vi "validate_ManipJump_v0.01.vi"(0 "Start Position":T3(ring), 1 "which manipulator":T5(ring), 2 "valve Time Cluster":T2, 3 "data in":T4={"daq_ao 1"="Dev1/ao0", "daq_ai 1"="Dev1/ai0", "experiment day folder"=path "D:/DATA/8-27-15 save func testing/test.lvm", "Multiclamp init error"=0, "Multiclamp Handle Out"=0, "sampling rate (Hz)"=10000, "trial name"=""}, 5 "Jump Position":T3(ring), 7 "controls array in":refnum<vi>[](array[refnum]), 9 "time to wait for solution change (min)":dbl=2.5 min=0.0 step=0.01, 11 "error in":errorcluster, 12 "common cluster":T7, 13 "individual controls in":T6) -> (4 "output cluster":T1={"daq_ao 2"="", "Duration (s)"=0.0, "Sample Freq (Hz)"=0.0, "Phase"=0.0, "Duty Cycle"=0.0, "Jump Filter Freq (Hz)"=0.0, "Number of Replicates"=1} {"Number of Replicates" min=1 max=10}, 6 "protocol waveform":waveform(dbl)(graph), 8 "protocol response":waveform(dbl)[](graph) caption="protcol response", 10 "control array out":refnum<vi>[](array[refnum]), 15 "error out":errorcluster)   [LabVIEW 2019]
uses:
  controls/scope_motion.ctl
  pipette cleaning/pressure box/cleaning_soft/controls/actuator_type.ctl
  pipette cleaning/pressure box/cleaning_soft/controls/actuator_cluster.ctl
  machine_vision/coordinate model vis/transform_properties_actuators.ctl
  machine_vision/controls/transform_cluster_actuator.ctl
  controls/NH_method.ctl
  pipette cleaning/pressure box/cleaning_soft/controls/pressure_box_type.ctl
  pipette cleaning/pressure box/cleaning_soft/controls/pressure_box_control.ctl
  multipatch/controls/multipatch_common_controls_v4.ctl
  controls/memtest_def.ctl
  multipatch/controls/multipatch_individual_controls_v5.ctl
  Controls/Data.ctl
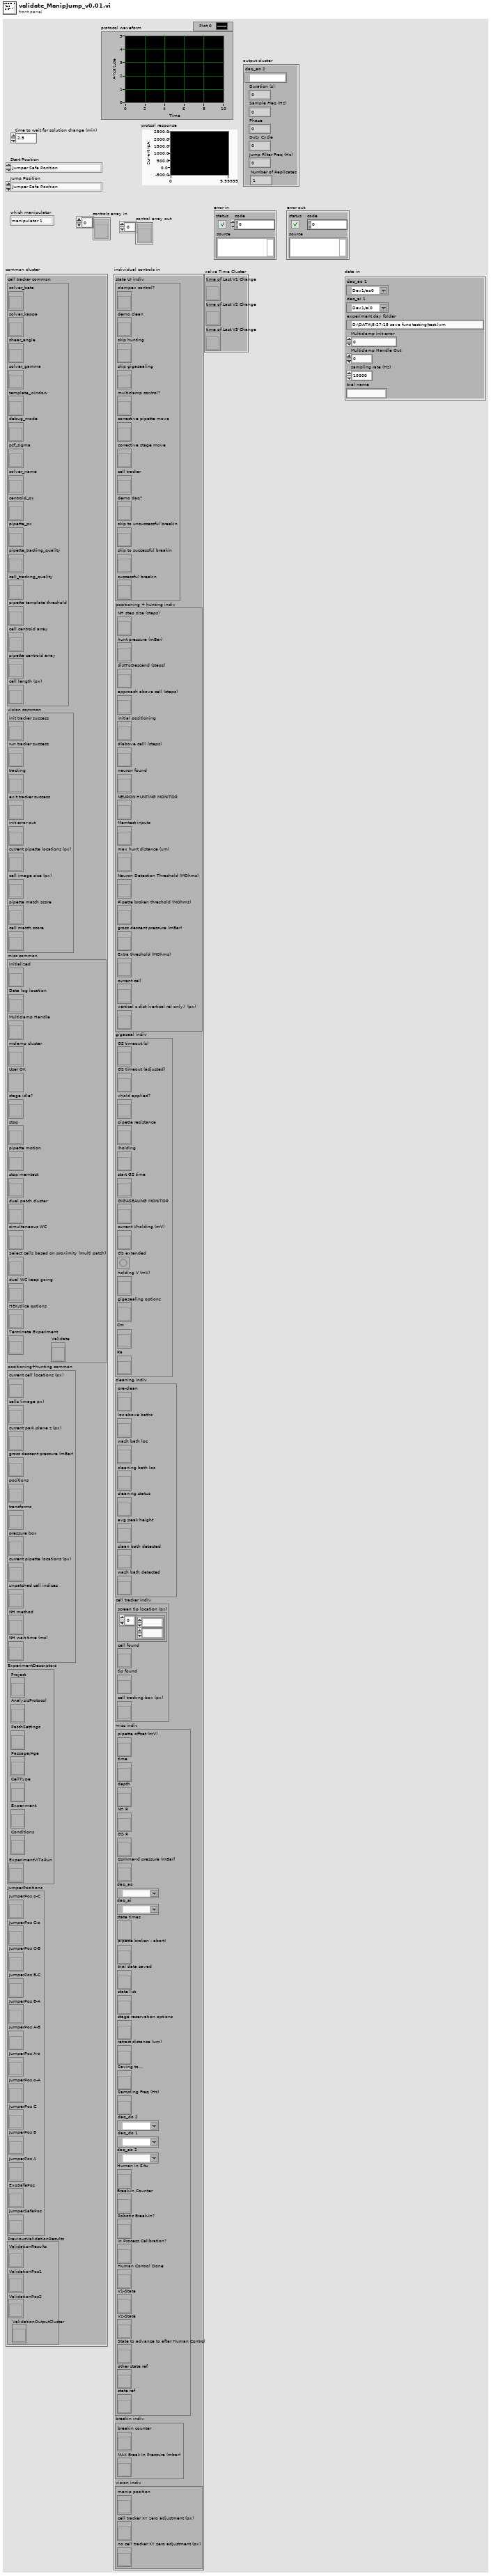
[diagram p1: front panel]
types:
  T1 = cluster{"daq_ao 2":tag, "Duration (s)":dbl, "Sample Freq (Hz)":dbl, "Phase":dbl, "Duty Cycle":dbl, "Jump Filter Freq (Hz)":dbl, "Number of Replicates":i16}
  T2 = cluster{"time of Last V1 Change":refnum<vi>, "time of Last V2 Change":refnum<vi>, "time of Last V3 Change":refnum<vi>}
  T3 = enum16{"Jumper Safe Position", "Experiment Safe Position", "Jumper Position A", "Jumper Position B", "Jumper Position C", "Jumper Position o-A", "Jumper Position A-o", "Jumper Position A-B", "Jumper Position B-A", "Jumper Position B-C", "Jumper Position C-B", "Jumper Position C-o", "Jumper Position o-C"}
  T4 = typedef "Data.ctl" = cluster{"daq_ao 1":tag, "daq_ai 1":tag, "experiment day folder":path, "Multiclamp init error":i32, "Multiclamp Handle Out":u32, "sampling rate (Hz)":i32, "trial name":string}
  T5 = enum16{"manipulator 1", "manipulator 2", "manipulator 3", "manipulator 4"}
  T6 = typedef "multipatch_individual_controls_v5.ctl" = cluster{"state UI indiv":cluster{"clampex control?":refnum<vi>, "demo clean":refnum<vi>, "skip hunting":refnum<vi>, "skip gigasealing":refnum<vi>, "multiclamp control?":refnum<vi>, "corrective pipette move":refnum<vi>, "corrective stage move":refnum<vi>, "cell tracker":refnum<vi>, "demo daq?":refnum<vi>, "skip to unsuccessful breakin":refnum<vi>, "skip to successful breakin":refnum<vi>, "successful breakin":refnum<vi>}, "positioning + hunting indiv":cluster{"NH step size (steps)":refnum<vi>, "hunt pressure (mBar)":refnum<vi>, "distToDescend (steps)":refnum<vi>, "approach above cell (steps)":refnum<vi>, "initial positioning":refnum<vi>, "d(above cell) (steps)":refnum<vi>, "neuron found":refnum<vi>, "NEURON HUNTING MONITOR":refnum<vi>, "Memtest inputs":refnum<vi>, "max hunt distance (um)":refnum<vi>, "Neuron Detection Threshold (MOhms)":refnum<vi>, "Pipette broken threshold (MOhms)":refnum<vi>, "gross descent pressure (mBar)":refnum<vi>, "Extra threshold (MOhms)":refnum<vi>, "current cell":refnum<vi>, "vertical z dist (vertical rel only)  (px)":refnum<vi>}, "gigaseal indiv":cluster{"GS timeout (s)":refnum<vi>, "GS timeout (adjusted)":refnum<vi>, "vhold applied?":refnum<vi>, "pipette resistance":refnum<vi>, "Iholding":refnum<vi>, "start GS time":refnum<vi>, "GIGASEALING MONITOR":refnum<vi>, "current Vholding (mV)":refnum<vi>, "GS extended":refnum<vi>, "holding V (mV)":refnum<vi>, "gigasealing options":refnum<vi>, "Cm":refnum<vi>, "Ra ":refnum<vi>}, "cleaning indiv":cluster{"pre-clean":refnum<vi>, "loc above baths":refnum<vi>, "wash bath loc":refnum<vi>, "cleaning bath loc":refnum<vi>, "cleaning status":refnum<vi>, "avg peak height":refnum<vi>, "clean bath detected":refnum<vi>, "wash bath detected":refnum<vi>}, "cell tracker indiv":cluster{"screen tip location (px)":refnum<vi>, "cell found":refnum<vi>, "tip found":refnum<vi>, "cell tracking box (px)":refnum<vi>}, "misc indiv":cluster{"pipette offset (mV)":refnum<vi>, "time":refnum<vi>, "depth":refnum<vi>, "NH R":refnum<vi>, "GS R":refnum<vi>, "Command pressure (mBar)":refnum<vi>, "daq_ao":tag, "daq_ai":tag, "state times":refnum<vi>, "pipette broken - abort!":refnum<vi>, "trial data saved":refnum<vi>, "state list":refnum<vi>, "stage reservation options":refnum<vi>, "retract distance (um)":refnum<vi>, "Saving to...":refnum<vi>, "Sampling Freq (Hz)":refnum<vi>, "daq_do 2":tag, "daq_do 1":tag, "daq_ao 2":tag, "Human in Situ":refnum<vi>, "Break-In Counter":refnum<vi>, "Robotic Break-In?":refnum<vi>, "In Process Calibration?":refnum<vi>, "Human Control Done":refnum<vi>, "V1-State":refnum<vi>, "V2-State":refnum<vi>, "State to advance to after Human Control":refnum<vi>, "other state ref":refnum<vi>, "state ref":refnum<vi>}, "breakin indiv":cluster{"breakin counter":refnum<vi>, "MAX Break In Pressure (mbar)":refnum<vi>}, "vision indiv":cluster{"manip position":refnum<vi>, "cell tracker XY zero adjustment (px)":refnum<vi>, "no cell tracker XY zero adjustment (px)":refnum<vi>}}
  T7 = typedef "multipatch_common_controls_v4.ctl" = cluster{"cell tracker common":cluster{"solver_beta":refnum<vi>, "solver_kappa":refnum<vi>, "shear_angle":refnum<vi>, "solver_gamma":refnum<vi>, "template_window":refnum<vi>, "debug_mode":refnum<vi>, "psf_sigma":refnum<vi>, "solver_name":refnum<vi>, "centroid_px":refnum<vi>, "pipette_px":refnum<vi>, "pipette_tracking_quality":refnum<vi>, "cell_tracking_quality":refnum<vi>, "pipette template threshold":refnum<vi>, "cell centroid array":refnum<vi>, "pipette centroid array":refnum<vi>, "cell length (px)":refnum<vi>}, "vision common":cluster{"init tracker success":refnum<vi>, "run tracker success":refnum<vi>, "tracking":refnum<vi>, "exit tracker success":refnum<vi>, "init error out":refnum<vi>, "current pipette locations (px)":refnum<vi>, "cell image size (px)":refnum<vi>, "pipette match score":refnum<vi>, "cell match score":refnum<vi>}, "misc common":cluster{"initialized":refnum<vi>, "Data log location":refnum<vi>, "Multiclamp Handle":refnum<vi>, "mclamp cluster":refnum<vi>, "User OK":refnum<vi>, "stage idle?":refnum<vi>, "stop":refnum<vi>, "pipette motion":refnum<vi>, "stop memtest":refnum<vi>, "dual patch cluster":refnum<vi>, "simultaneous WC":refnum<vi>, "Select cells based on proximity (multi patch)":refnum<vi>, "dual WC keep going":refnum<vi>, "HEK/slice options":refnum<vi>, "Terminate Experiment":refnum<vi>, "Validate":refnum<vi>}, "positioning+hunting common":cluster{"current cell locations (px)":refnum<vi>, "cells (image px)":refnum<vi>, "current park plane z (px)":refnum<vi>, "gross descent pressure (mBar)":refnum<vi>, "positions":refnum<vi>, "transforms":refnum<vi>, "pressure box":refnum<vi>, "current pipette locations (px)":refnum<vi>, "unpatched cell indices":refnum<vi>, "NH method":refnum<vi>, "NH wait time (ms)":refnum<vi>}, "ExperimentDescriptors":cluster{"Project":refnum<vi>, "AnalysisProtocol":refnum<vi>, "PatchSettings":refnum<vi>, "Passage/Age":refnum<vi>, "CellType":refnum<vi>, "Experiment":refnum<vi>, "Conditions":refnum<vi>, "ExperimentVIToRun":refnum<vi>}, "JumperPositions":cluster{"JumperPos o-C":refnum<vi>, "JumperPos C-o":refnum<vi>, "JumperPos C-B":refnum<vi>, "JumperPos B-C":refnum<vi>, "JumperPos B-A":refnum<vi>, "JumperPos A-B":refnum<vi>, "JumperPos A-o":refnum<vi>, "JumperPos o-A":refnum<vi>, "JumperPos C":refnum<vi>, "JumperPos B":refnum<vi>, "JumperPos A":refnum<vi>, "ExpSafePos":refnum<vi>, "jumperSafePos":refnum<vi>}, "PreviousValidationResults":cluster{"ValidationResults":refnum<vi>, "ValidationPos1":refnum<vi>, "ValidationPos2":refnum<vi>, "ValidationOutputCluster":refnum<vi>}}
  T8 = typedef "transform_cluster_actuator.ctl" = cluster{"s":refnum<vi>, "manip 1":refnum<vi>, "manip 2":refnum<vi>, "manip 3":refnum<vi>, "manip 4":refnum<vi>}
  T9 = typedef "scope_motion.ctl" = enum16{"superSlow", "fast", "slow", "find slice speed", "slow_dualPatch"}
  T10 = typedef "transform_properties_actuators.ctl" = cluster{"theta (deg)":dbl, "X sc factor (px/step)":dbl, "Y sc factor (px/step)":dbl, "zero loc (x,y,z)":dbl[], "flip y?":bool, "flip x?":bool, "gamma (deg)":dbl, "flip z?":bool, "Z sc factor (px/step)":dbl, "actuator":T11, "safe space (steps)":i32[]}
  T11 = typedef "actuator_cluster.ctl" = cluster{"Actuator COM":refnum<visa-resource-name>, "Actuator type":T12}
  T12 = typedef "actuator_type.ctl" = enum16{"Scientifica", "Sutter", "Demo", "Off"}
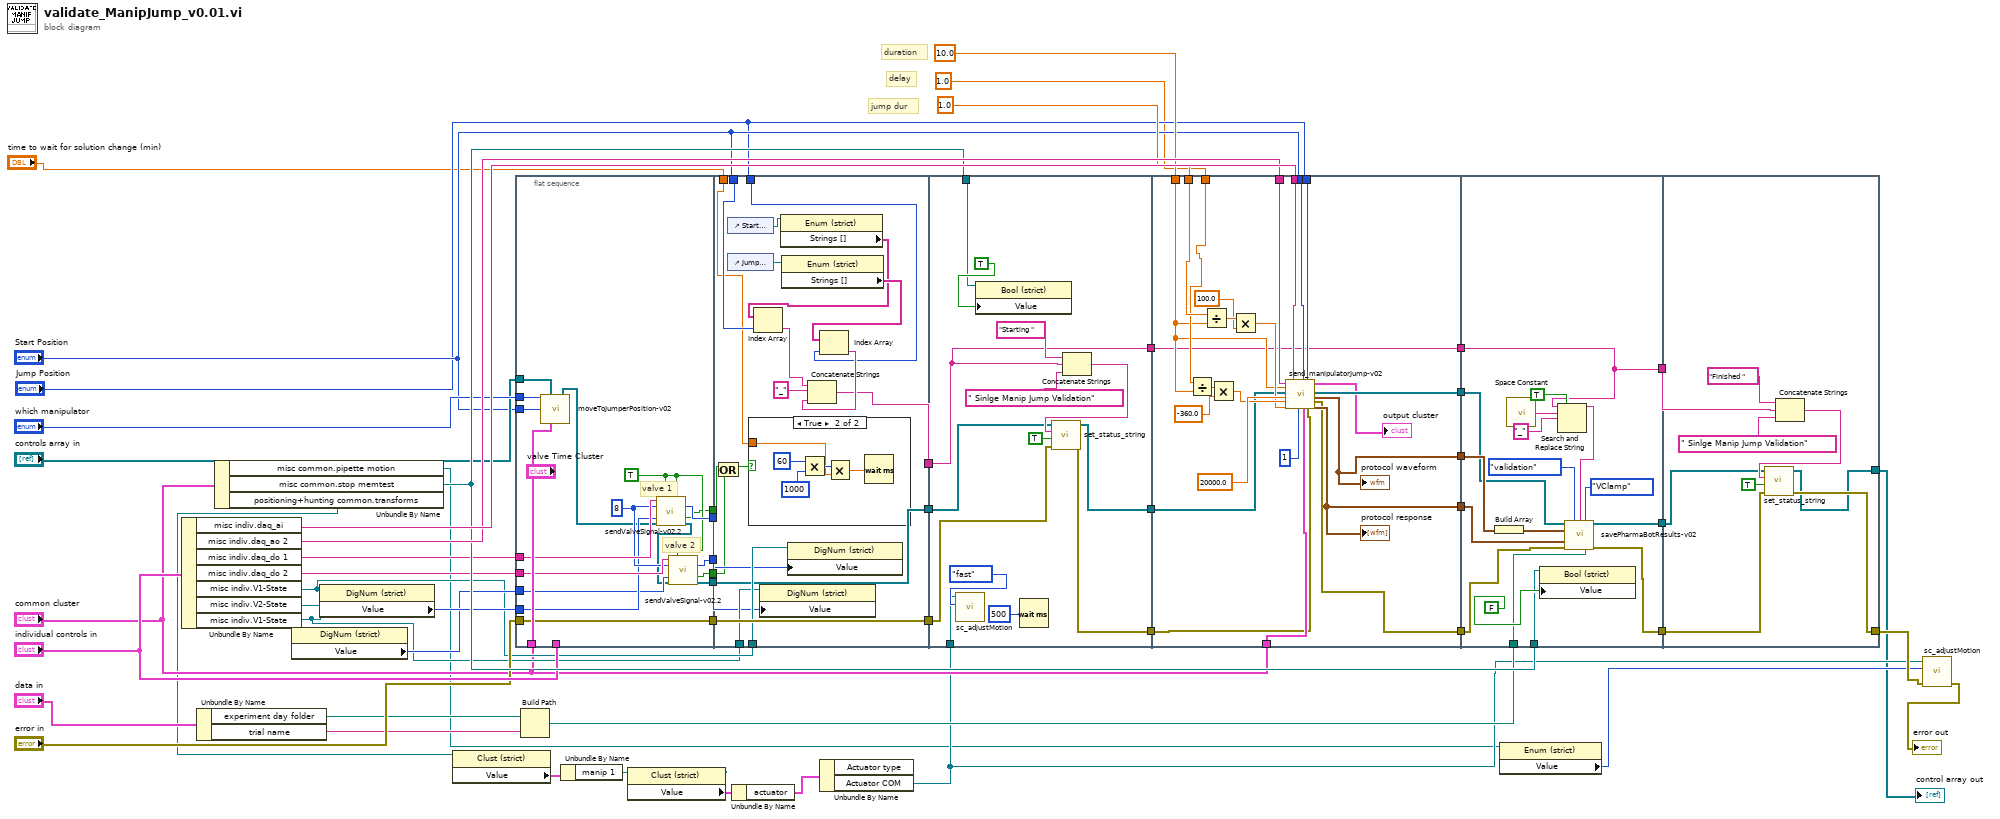
[diagram p0: block diagram]
diagram:
  # "jump dur"
  # "delay"
  # "duration"
  n1 = Unbundle By Name("individual controls in") -> ("misc indiv.daq_ai"=w55:tag, "misc indiv.daq_ao 2"=w54:tag, "misc indiv.daq_do 1"=w50:tag, "misc indiv.daq_do 2"=w49:tag, "misc indiv.V1-State"=w41:refnum<vi>, "misc indiv.V2-State"=w40:refnum<vi>)  [unwired: 1 out]
  n2 = Unbundle By Name("data in") -> ("experiment day folder"=w34:path, "trial name"=w33:string)
  n3 = Unbundle By Name("common cluster") -> ("misc common.pipette motion"=w21:refnum<vi>, "misc common.stop memtest"=w53:refnum<vi>, "positioning+hunting common.transforms"=w28:refnum<vi>)
  n4 = property class="DigNum (strict)"(reference=w40) -> ("Value"=w42:u16)  [unwired: 1 in, 2 out]
  n5 = property class="DigNum (strict)"(reference=w41) -> ("Value"=w43:u16)  [unwired: 1 in, 2 out]
  n6 = property class="Clust (strict)"(reference=w28) -> ("Value"=w29:T8)  [unwired: 1 in, 2 out]
  n7 = flat-sequence {
    tunnel: "which manipulator" -> [w73]
    tunnel: "Start Position" -> [w72]
    tunnel: "common cluster" -> [w71]
    tunnel: "individual controls in" -> [_]
    tunnel: w50 -> [w70]
    tunnel: w49 -> [w69]
    tunnel: "error in" -> [w67]
    tunnel: [w67] -> w44
    tunnel: w43 -> [w66]
    tunnel: w42 -> [w65]
    tunnel: [w64] -> w39
    tunnel: [w63] -> w38
    tunnel: "controls array in" -> [w62]
    tunnel: [w59] -> w15
    tunnel: [w57] -> w3
    tunnel: [w56] -> w2
    tunnel: [w93] -> w45
    tunnel: w44 -> [w93]
    tunnel: w41 -> [w92]
    tunnel: w40 -> [w91]
    tunnel: w39 -> [w90]
    tunnel: w38 -> [w89]
    tunnel: [w88] -> w16
    tunnel: w15 -> [w88]
    tunnel: "Start Position" -> [w80]
    tunnel: "Jump Position" -> [w79]
    tunnel: [w78] -> w7
    tunnel: w3 -> [w76]
    tunnel: w2 -> [w75]
    tunnel: "time to wait for solution change (min)" -> [w74]
    tunnel: w53 -> [w110]
    tunnel: [w99] -> w46
    tunnel: w45 -> [w100]
    tunnel: w23 -> [w108]
    tunnel: w16 -> [w102]
    tunnel: [w101] -> w14
    tunnel: w7 -> [w103]
    tunnel: [w103] -> w5
    tunnel: w55 -> [w135]
    tunnel: w54 -> [w134]
    tunnel: [w118] -> w47
    tunnel: w46 -> [w119]
    tunnel: [w114] -> w37
    tunnel: [w133] -> w36
    tunnel: "common cluster" -> [w120]
    tunnel: "Start Position" -> [w132]
    tunnel: "Jump Position" -> [w131]
    tunnel: 10.0 ("Duration (s)") -> [w121]
    tunnel: 1.0 ("Jump Duration (s)") -> [w126]
    tunnel: 1.0 ("Jump Delay (s)") -> [w125]
    tunnel: w14 -> [w117]
    tunnel: [w116] -> w13
    tunnel: [w115] -> w6
    tunnel: w5 -> [w115]
    tunnel: w53 -> [w152]
    tunnel: w47 -> [w141]
    tunnel: w37 -> [w151]
    tunnel: w36 -> [w149]
    tunnel: w32 -> [w146]
    tunnel: [w137] -> w18
    tunnel: w13 -> [w140]
    tunnel: [w139] -> w12
    tunnel: [w138] -> w10
    tunnel: w6 -> [w138]
    tunnel: [w157] -> w25
    tunnel: w18 -> [w158]
    tunnel: w12 -> [w159]
    tunnel: [w156] -> w11
    tunnel: w10 -> [w155]
    frame #0 {
      w58 = TRUE ("Set Status")
      w68 = u16 8 ("ChangeToValve")
      # "valve 2"
      # "valve 1"
      n8 = call "moveToJumperPosition-v02.vi"("which manipulator"=w73, "controls array in"=w62, "Which Jumper Position to move to?"=w72, "common cluster"=w71) -> ("control array out"=w61:refnum<vi>[])  [unwired: 10 in, 1 out]
      n9 = call "sendValveSignal-v02.2.vi"("daq_do"=w70, "Valve1?"=w58, "ChangeToValve"=w68, "CurrentValve"=w66, "controls array in"=w61, "Set Status"=w58) -> ("ValveSetTo"=w63:u16, "valve changed?"=w57:bool, "control array out"=w60:refnum<vi>[])  [unwired: 6 in, 1 out]
      n10 = call "sendValveSignal-v02.2.vi"("daq_do"=w69, "ChangeToValve"=w68, "CurrentValve"=w65, "controls array in"=w60, "Set Status"=w58) -> ("ValveSetTo"=w64:u16, "valve changed?"=w56:bool, "control array out"=w59:refnum<vi>[])  [unwired: 7 in, 1 out]
    }
    frame #1 {
      n11 = Or(x=w76, y=w75) -> (x .or. y?=w77:bool)
      n12 = control-ref of="Start Position"() -> (w82:refnum<vi>)
      n13 = control-ref of="Jump Position"() -> (w83:refnum<vi>)
      n14 = case shown="True" w77 {
        tunnel: w74 -> [_ w94]
        frame False {
        }
        frame True {
          n15 = Multiply(x=u32 60 ("milliseconds to wait"), y=u32 1000) -> (x*y=w96:u32)
          n16 = Multiply(x=w96, y=w94) -> (x*y=w95:dbl)
          n17 = Wait (ms)(milliseconds to wait=w95) -> ()  [unwired: 1 out]
        }
      }
      n18 = property class="DigNum (strict)"(reference=w91, "Value"=w90) -> ()  [unwired: 1 in, 2 out]
      n19 = property class="Enum (strict)"(reference=w82) -> ("Strings []"=w86:string[])  [unwired: 1 in, 2 out]
      n20 = Index Array(array=w86, index=w80) -> (element=w85:string)
      n21 = property class="Enum (strict)"(reference=w83) -> ("Strings []"=w87:string[])  [unwired: 1 in, 2 out]
      n22 = property class="DigNum (strict)"(reference=w92, "Value"=w89) -> ()  [unwired: 1 in, 2 out]
      n23 = Index Array(array=w87, index=w79) -> (element=w81:string)
      n24 = Concatenate Strings(w85, "_", w81) -> (w78:string)
    }
    frame #2 {
      n25 = call "sc_adjustMotion.vi"("motion"=scope_motion."fast", "VISA handle"=w108) -> ()  [unwired: 8 in, 2 out]
      n26 = property class="Bool (strict)"(reference=w110, "Value"=TRUE ("stop memtest")) -> ()  [unwired: 1 in, 2 out]
      n27 = Wait (ms)(milliseconds to wait=u32 500) -> ()  [unwired: 1 out]
      n28 = Concatenate Strings("Starting " ("string"), w103, " Sinlge Manip Jump Validation" ("string")) -> (w106:string)
      n29 = call "set_status_string.vi"("error in"=w100, "new line?"=TRUE, "status string in"=w106, "controls array"=w102) -> ("error out"=w99:errorcluster, "controls array out"=w101:refnum<vi>[])  [unwired: 6 in]
    }
    frame #3 {
      n30 = Divide(x=w125, y=w121) -> (x/y=w127:dbl)
      n31 = Divide(x=w126, y=w121) -> (x/y=w130:dbl)
      n32 = Multiply(x=w127, y=-360.0) -> (x*y=w124:dbl)
      n33 = Multiply(x=w130, y=100.0) -> (x*y=w123:dbl)
      n34 = call "send_manipulatorJump-v02.vi"("daq_ao 2"=w134, "Duration (s)"=w121, "controls array in"=w117, "Sample Freq (Hz)"=20000.0, "Phase"=w124, "Duty Cycle"=w123, "daq_ai"=w135, "Number of Replicates"=i16 1, "Start Position"=w132, "common cluster"=w120, "Jump Position"=w131, "error in"=w119) -> ("output cluster"=→"output cluster":T1, "control array out"=w116:refnum<vi>[], "protcol waveform"=w114:waveform(dbl), "error out"=w118:errorcluster, "protcol response"=w133:waveform(dbl)[])  [unwired: 3 in]
      "protocol response" <- w133
      "protocol waveform" <- w114
    }
    frame #4 {
      n35 = Build Array(w151) -> (w150:waveform(dbl)[])
      n36 = call <vilib>:"Space Constant.vi"() -> ("String"=w144:string)
      n37 = property class="Bool (strict)"(reference=w152, "Value"=FALSE ("stop memtest")) -> ()  [unwired: 1 in, 2 out]
      n38 = Search and Replace String(replace all?=TRUE ("replace all? (F)"), input string=w138, search string=w144, replace string="_" ("replace string (\"\")")) -> (result string=w142:string)  [unwired: 4 in, 3 out]
      n39 = call "savePharmaBotResults-v02.vi"("controls array"=w140, "protocol or memtest"=enum16{"protocol", "memtest", "validation"}."validation", "ExpPhase"=w142, "which clamp"=enum16{"VClamp", "IClamp"}."VClamp", "protocol waveform"=w150, "protocol response"=w149, "error in"=w141, "Save to (folder dir)"=w146) -> ("controls array out"=w139:refnum<vi>[], "error out"=w137:errorcluster)  [unwired: 6 in]
    }
    frame #5 {
      n40 = Concatenate Strings("Finished " ("string"), w155, " Sinlge Manip Jump Validation" ("string")) -> (w161:string)
      n41 = call "set_status_string.vi"("error in"=w158, "new line?"=TRUE, "status string in"=w161, "controls array"=w159) -> ("error out"=w157:errorcluster, "controls array out"=w156:refnum<vi>[])  [unwired: 6 in]
    }
  }
  n42 = Build Path(base path=w34, name or relative path=w33) -> (appended path=w32:path)
  n43 = Unbundle By Name(w29) -> ("manip 1"=w30:refnum<vi>)
  n44 = property class="Clust (strict)"(reference=w30) -> ("Value"=w27:T10)  [unwired: 1 in, 2 out]
  n45 = Unbundle By Name(w27) -> ("actuator"=w26:T11)
  n46 = Unbundle By Name(w26) -> ("Actuator COM"=w23:refnum<visa-resource-name>)  [unwired: 1 out]
  n47 = property class="Enum (strict)"(reference=w21) -> ("Value"=w22:T9)  [unwired: 1 in, 2 out]
  n48 = call "sc_adjustMotion.vi"("error in (no error)"=w25, "motion"=w22, "VISA handle"=w23) -> ("error out"=→"error out":errorcluster)  [unwired: 7 in, 1 out]
  "control array out" <- w11
